vi "SwerveKinematics_New4.vi"(8 "wheel 3":T3 {"Y" format="%14.3f"; "X" format="%14.3f"}, 9 "wheel 2":T3 {"Y" format="%14.3f"; "X" format="%14.3f"}, 10 "wheel 1":T3 {"Y" format="%14.3f"; "X" format="%14.3f"}, 11 "wheel 0":T3 {"Y" format="%14.3f"; "X" format="%14.3f"}) -> (3 "SWERVE_DRIVE_KINEMATICS":T1 {"PrevCoR"."Y" format="%14.3f"; "PrevCoR"."X" format="%14.3f"; "Modules"."Y" format="%14.3f"; "Modules"."X" format="%14.3f"})   [LabVIEW 2019, in "Trajectory_Library.lvlib"]
doc: "Constructs a swerve drive kinematics object. This takes in a variable number of wheel locations as Translation2ds. The order in which you pass in the wheel locations is the same order that you will recieve the module states when performing inverse kinematics. It is also expected that you pass in the module states in the same order when calling the forward kinematics methods. This subVI is customized for 4 wheel modules.\n\nThis is a helper class that converts a chassis velocity (dx, dy, and dtheta components) into individual module states (speed and angle).\n \nThe inverse kinematics (converting from a desired chassis velocity to individual module states) uses the relative locations of the modules with respect to the center of rotation. The center of rotation for inverse kinematics is also variable. This means that you can set your set your center of rotation in a corner of the robot to perform special evasion manuevers.\n \nForward kinematics (converting an array of module states into the overall chassis motion) is performs the exact opposite of what inverse kinematics does. Since this is an overdetermined system (more equations than variables), we use a least-squares approximation.\n \nThe inverse kinematics: [moduleStates] = [moduleLocations][chassisSpeeds] We take the Moore-Penrose pseudoinverse of [moduleLocations] and then multiply by [moduleStates] to get our chassis speeds.\n \nForward kinematics is also used for odometry -- determining the position of the robot on the field using encoders and a gyro.\n\nParameters: \n - wheel 0 - Translation data structures indicating the location of a wheel relative to the physical center of the robot.\n - wheel 1 - Translation data structures indicating the location of a wheel relative to the physical center of the robot. (Meters)\n - wheel 2 - Translation data structures indicating the location of a wheel relative to the physical center of the robot. (Meters)\n - wheel 3 - Translation data structures indicating the location of a wheel relative to the physical center of the robot. (Meters)\n\nReturns:\n - SwerveDriveKinematics - The initialized data structure"
uses:
  Trajectory_Library.lvlib
  TypeDef/TRANSLATION2D.ctl
  TypeDef/SWERVE_DRIVE_KINEMATICS.ctl
  <vilib>/Analysis/Matrix/Datatypes/RealMatrix.ctl
  <vilib>/Analysis/Matrix/NI_Matrix.lvlib
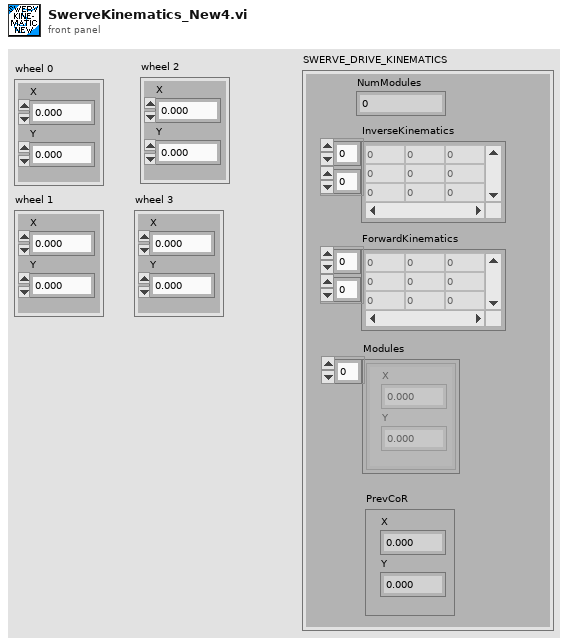
[diagram p1: front panel]
types:
  T1 = typedef "Trajectory_Library.lvlib/SWERVE_DRIVE_KINEMATICS.ctl" = cluster{"NumModules":i32, "InverseKinematics":T2, "ForwardKinematics":T2, "Modules":T3[], "PrevCoR":T3}
  T2 = typedef "NI_Matrix.lvlib/RealMatrix.ctl" = dbl[][]
  T3 = typedef "Trajectory_Library.lvlib/TRANSLATION2D.ctl" = cluster{"X":dbl, "Y":dbl}
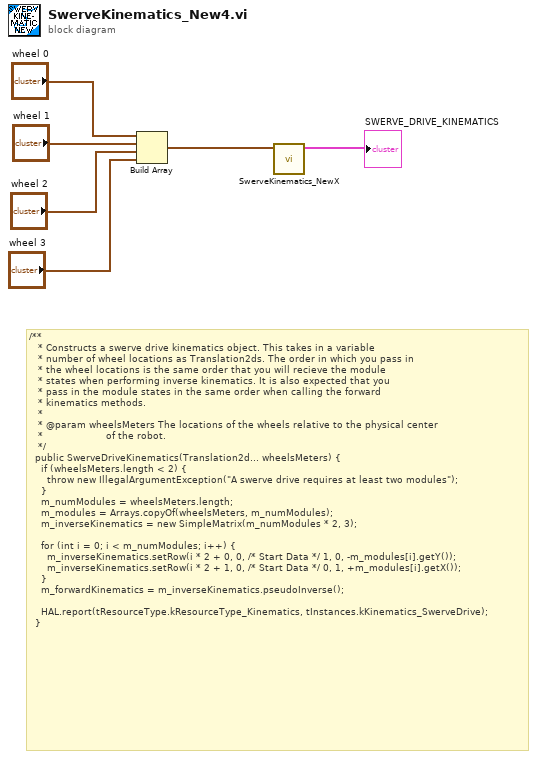
[diagram p0: block diagram]
diagram:
  # "/**\n   * Constructs a swerve drive kinematics object. This takes in a variable\n   * number of wheel locations as Translation2ds. The order in which you pass in\n   * the wheel locations is the same order that you will recieve the module\n   * states when performing inverse kinematics. It is also expected that you\n   * pass in the module states in the same order when calling the forward\n   * kinematics methods.\n   *\n   * @param wheelsMeters The locations of the wheels relative to the physical center\n   *                     of the robot.\n   */\n  public SwerveDriveKinematics(Translation2d... wheelsMeters) {\n    if (wheelsMeters.length < 2) {\n      throw new IllegalArgumentException(\"A swerve drive requires at least two modules\");\n    }\n    m_numModules = wheelsMeters.length;\n    m_modules = Arrays.copyOf(wheelsMeters, m_numModules);\n    m_inverseKinematics = new SimpleMatrix(m_numModules * 2, 3);\n\n    for (int i = 0; i < m_numModules; i++) {\n      m_inverseKinematics.setRow(i * 2 + 0, 0, /* Start Data */ 1, 0, -m_modules[i].getY());\n      m_inverseKinematics.setRow(i * 2 + 1, 0, /* Start Data */ 0, 1, +m_modules[i].getX());\n    }\n    m_forwardKinematics = m_inverseKinematics.pseudoInverse();\n\n    HAL.report(tResourceType.kResourceType_Kinematics, tInstances.kKinematics_SwerveDrive);\n  }"
  n1 = Build Array("wheel 0", "wheel 1", "wheel 2", "wheel 3") -> (w2:T3[])
  n2 = call "SwerveKinematics_NewX.vi"("Wheels"=w2) -> ("SWERVE_DRIVE_KINEMATICS"=→"SWERVE_DRIVE_KINEMATICS":T1)  [unwired: 10 in]
